vi "Parse.vi"(8 "error in":errorcluster, 11 "String":string) -> (0 "error out":errorcluster)   [LabVIEW 2015, in "TCP.lvlib"]
uses:
  TCP.lvlib
  support/Message Queue/Enqueue Message (Single).vi
  support/Message Queue/Message Queue.lvlib
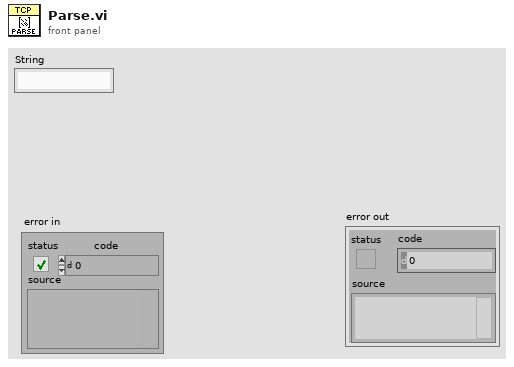
[diagram p1: front panel]
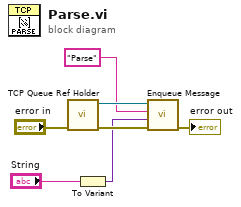
[diagram p0: block diagram]
diagram:
  n1 = call "TCP Queue Ref Holder.vi"("error in"="error in") -> ("error out"=w6:errorcluster, "Input Message Queue"=w4:refnum<queue>)  [unwired: 9 in]
  n2 = To Variant(anything="String") -> (Variant=w1:variant)
  n3 = call-poly "Enqueue Message.vi"("error in (no error)"=w6, "Message Data"=w1, "Message"="Parse", "Message Queue"=w4) -> ("error out"=→"error out":errorcluster)  [unwired: 6 in, 1 out]
